vi "ShowData.vi"(11 "data in":refnum<class "EventMessengerPData.lvclass">) -> (0 "aborted?":bool, 2 "write count":u32, 3 "data out":refnum<class "EventMessengerPData.lvclass">, 4 "last element?":bool)   [LabVIEW 2020, in "Event Messenger Priority.lvlib" / "EventMessengerPData.lvclass"]
uses:
  EventMessengerPData.lvclass
  EventMessengerPData.lvclass/EventMessengerPData.ctl
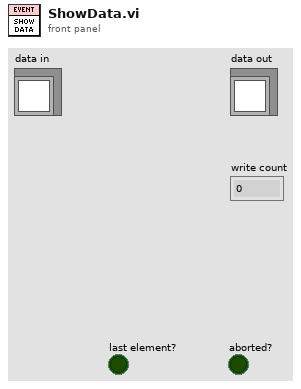
[diagram p1: front panel]
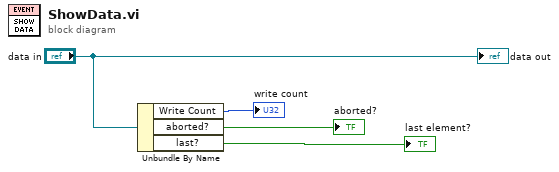
[diagram p0: block diagram]
diagram:
  n1 = Unbundle By Name("data in") -> ("Write Count"=→"write count":u32, "aborted?"=→"aborted?":bool, "last?"=→"last element?":bool)
  "data out" <- "data in"
